vi "Tx Ch Write.vi"(6 "pWritten":u32, 8 "pBuffer":u8[](array[numeric]), 9 "Length":u32, 10 "Channel":u8, 11 "devId":i32) -> (1 "devId out":i32, 3 "function return":i32, 4 "pWritten out":u32)   [LabVIEW 2013, in "CHR34XXX.lvlib"]
doc: "DLL BOOL __stdcall CHR34XXX_TxCh_SetMode(IN int devId,IN BYTE Channel,IN BYTE Mode); DLL BOOL __stdcall CHR34XXX_TxCh_SetPeriod(IN int devId,IN BYTE Channel,IN DWORD Period); DLL BOOL __stdcall CHR34XXX_TxCh_FIFOState(IN int devId,IN BYTE Channel,OUT DWORD *State); DLL BOOL __stdcall CHR34XXX_TxCh_FIFOCount(IN int devId,IN BYTE Channel,OUT DWORD *FIFOCount); DLL BOOL __stdcall CHR34XXX_TxCh_Write(IN int devId,IN BYTE Channel,IN DWORD Length,IN BYTE *pBuffer,OUT DWORD *pWritten);"
uses:
  CHR34XXX.lvlib
  CHR34XXX.dll
panel:
  out "pBuffer out":u8[](array[numeric])
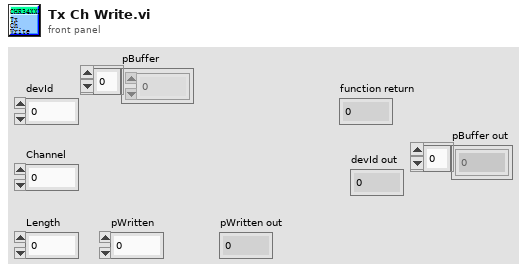
[diagram p1: front panel]
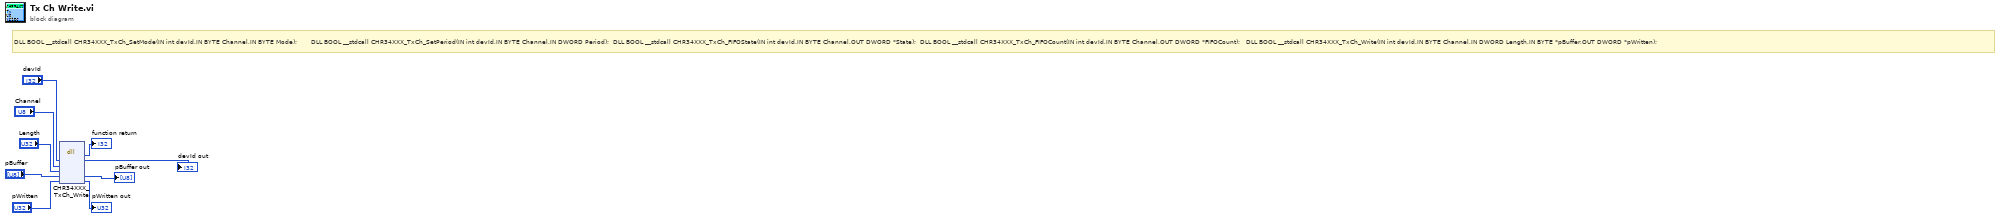
[diagram p0: block diagram]
diagram:
  # "DLL BOOL __stdcall CHR34XXX_TxCh_SetMode(IN int devId,IN BYTE Channel,IN BYTE Mode);       DLL BOOL __stdcall CHR34XXX_TxCh_SetPeriod(IN int devId,IN BYTE Channel,IN DWORD Period);  DLL BOOL __stdcall CHR34XXX_TxCh_FIFOState(IN int devId,IN BYTE Channel,OUT DWORD *State);  DLL BOOL __stdcall CHR34XXX_TxCh_FIFOCount(IN int devId,IN BYTE Channel,OUT DWORD *FIFOCount);   DLL BOOL __stdcall CHR34XXX_TxCh_Write(IN int devId,IN BYTE Channel,IN DWORD Length,IN BYTE *pBuffer,OUT DWORD *pWritten);"
  n1 = dll-call lib="C:/Users/dy/Desktop/CHR34XXX_lv/lv_lib/CHR34XXX.*" fn="CHR34XXX_TxCh_Write"("devId"="devId", "Channel"="Channel", "Length"="Length", "pBuffer"="pBuffer", "pWritten"="pWritten") -> ("返回类型"=→"function return":i32, "devId"=→"devId out":i32, "pBuffer"=→"pBuffer out":u8[], "pWritten"=→"pWritten out":u32)  [unwired: 5 in, 2 out]
